vi "Get SMO Public API.vi"(8 "error in (no error)":errorcluster, 11 "Inst.Framework-Template in":refnum<class "Inst.Framework-Template.lvclass">) -> (0 "error out":errorcluster, 2 "Commands":string[](array[string]), 3 "Inst.Framework-Template out":refnum<class "Inst.Framework-Template.lvclass">)   [LabVIEW 2019, in "Inst.Framework-Template.lvclass"]
uses:
  Inst.Framework-Template.lvclass
  Typedefs/Inst.Framework-Template.Commands--Enum.ctl
  <userlib>/LevyLab/Instrument Framework/Instrument Types/VSource/Instrument.VSource.lvclass
  <userlib>/LevyLab/Instrument Framework/SMOs/Instrument/Instrument.lvclass
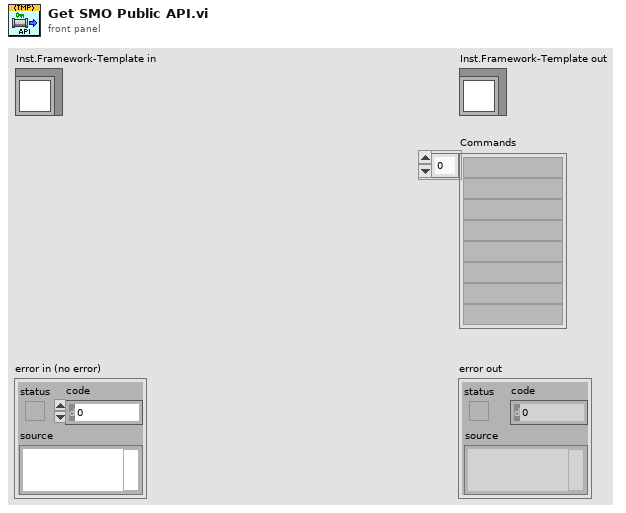
[diagram p1: front panel]
types:
  T1 = typedef "Inst.Framework-Template.lvclass/Inst.Framework-Template.Commands--Enum.ctl" = enum16{"Do Something"}
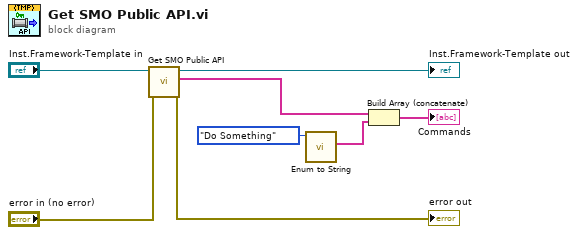
[diagram p0: block diagram]
diagram:
  n1 = call-parent "Get SMO Public API.vi"("error in (no error)"="error in (no error)", "Instrument in"="Inst.Framework-Template in") -> ("error out"=→"error out":errorcluster, "Commands"=w8:string[], "Instrument out"=→"Inst.Framework-Template out":refnum<class "Inst.Framework-Template.lvclass">)  [unwired: 7 in]
  n2 = call <userlib>:"Enum to String.vi"("Command"=Inst.Framework-Template.Commands--Enum."Do Something" ("Commands")) -> ("Commands []"=w3:string[])  [unwired: 9 in, 1 out]
  n3 = Build Array (concatenate)(w8, w3) -> (→"Commands":string[])
